vi "Auto-Fill.vi"() -> ()   [LabVIEW 2011]
uses:
  SubVI/Auto-Fill Cases.ctl
  SubVI/Valve_Pump.ctl
  SubVI/Pumps_Valves_Dependencies_Global.vi
panel:
  in  "Emergency Stop":bool
  out "Litres":dbl(slide) scale=0.0..14400.0
  out "Tank C":dbl(slide) scale=0.0..100.0
  out "Tank B":dbl(slide) scale=0.0..100.0
  out "Tank D":dbl(slide) scale=0.0..100.0
  out "Tank A":dbl(slide) scale=0.0..100.0
  in  "Density (kg/m3)":dbl[](array[numeric])=[0.0, 0.0, 0.0, 0.0, 0.0, 0.0]
  in  "Height (cm)":dbl[](array[numeric])=[0.0, 0.0, 0.0, 0.0, 0.0, 0.0]
  in  "Auto-Fill":T1
  in  "Start Process":bool
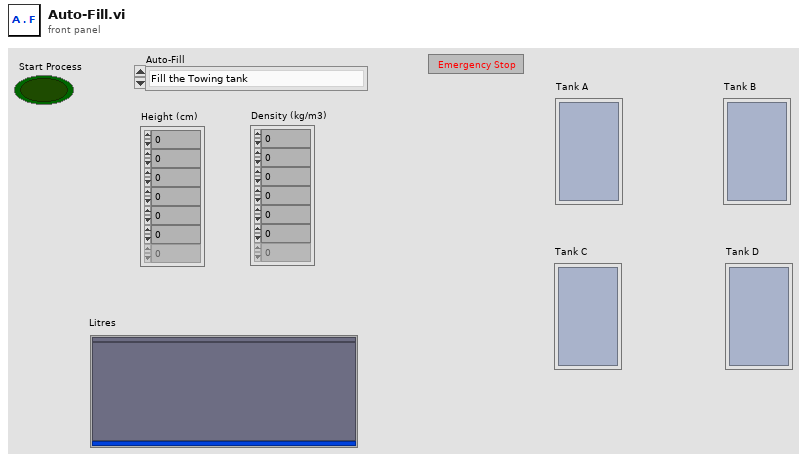
[diagram p1: front panel]
types:
  T1 = typedef "Auto-Fill Cases.ctl" = enum16{"Fill the Towing tank", "Fill Tank A from the Salt saturator tank", "Fill Tank B from the Salt Saturator tank", "Fill Tank C from the water mains", "Fill Tank D from the water mains", "Fill tank B from tank A", "Fill tank C from tank D"}
  T2 = typedef "Valve_Pump.ctl" = enum16{"Main Rack Power", "Pump Power", "Valve Power", "V4", "V5", "V6", "V7", "V8", "V9", "V10", "V11", "V12", "V13", "V14", "V15", "V18", "V19", "V20", "V21", "V22", "V23", "V24", "V25", "V26", "V27", "V28", "V29", "V30", "V31", "V32", "V33", "V34", "Pump A", "Pump B", "Pump C", "Pump D"}
  T3 = cluster{"Tanks[0]":dbl, "Tanks[1]":dbl, "Tanks[2]":dbl, "Tanks[3]":dbl, "Tanks[4]":dbl}
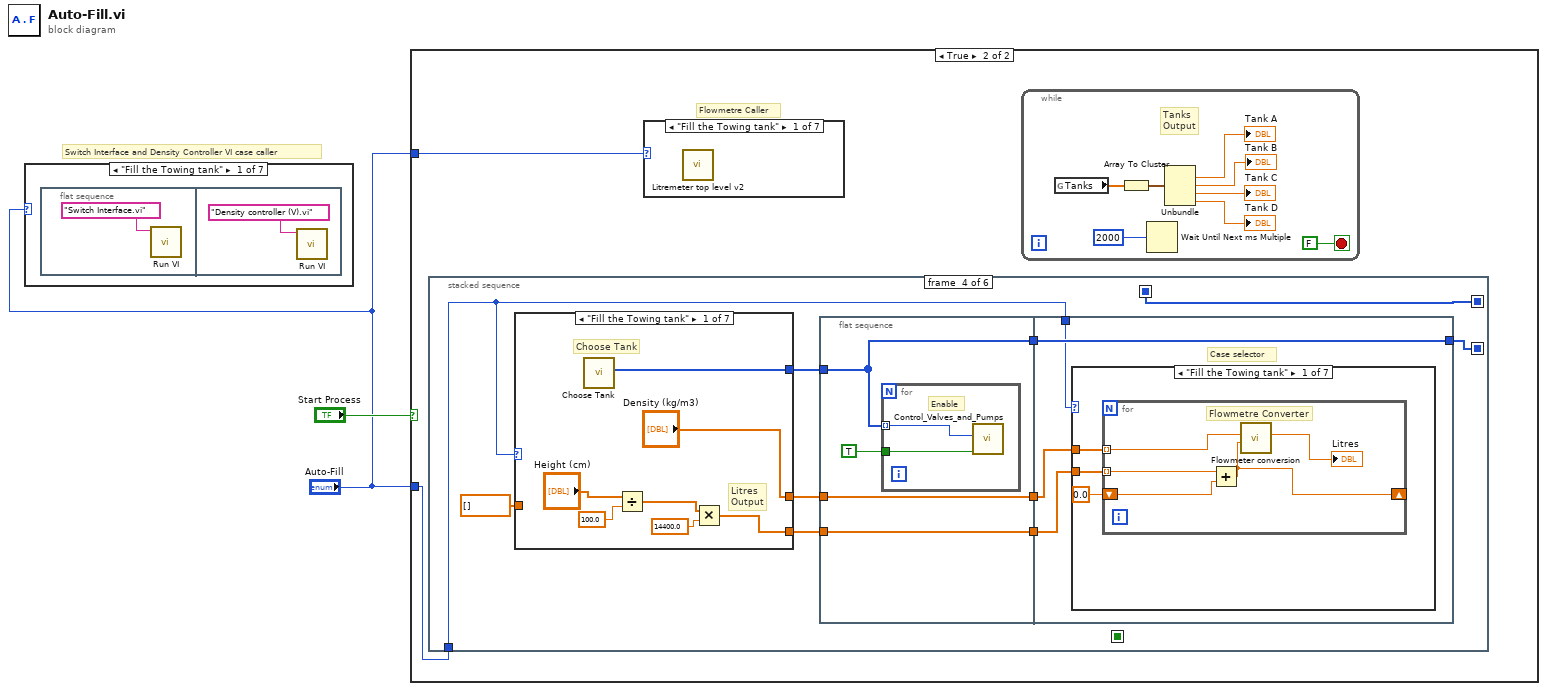
[diagram p0: block diagram]
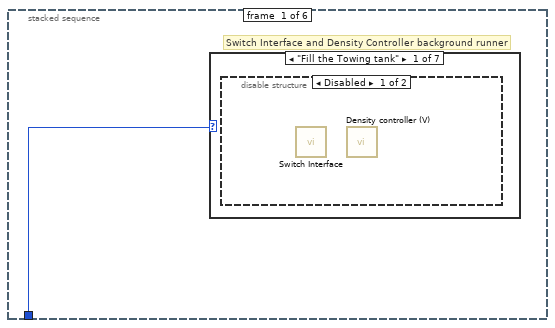
[diagram p15: hidden frame]
diagram:
  # "Switch Interface and Density Controller VI case caller"
  n1 = case shown="\"Fill the Towing tank\"" "Auto-Fill" {
    frame "Fill the Towing tank" {
      n2 = flat-sequence {
        frame #0 {
          n3 = call "Run VI.vi"("VI name"="Switch Interface.vi") -> ()  [unwired: 11 in]
        }
        frame #1 {
          n4 = call "Run VI.vi"("VI name"="Density controller (V).vi") -> ()  [unwired: 11 in]
        }
      }
    }
    frame "Fill Tank A from the Salt saturator tank" {
    }
    frame "Fill Tank B from the Salt Saturator tank" {
    }
    frame "Fill Tank C from the water mains" {
    }
    frame "Fill Tank D from the water mains" {
    }
    frame "Fill tank B from tank A" {
    }
    frame "Fill tank C from tank D" {
    }
  }
  n5 = case shown="True" "Start Process" {
    tunnel: "Auto-Fill" -> [_ w6]
    tunnel: "Auto-Fill" -> [_ w5]
    frame False {
    }
    frame True {
      # "Flowmetre Caller"
      n6 = stacked-sequence {
        seq-local: [_ _ w21 _ _ _] -> [_ _ _ w34 _ _]
        seq-local: [_ _ _ w31 _ _] -> [_ _ _ _ w141 _]
        seq-local: [_ _ _ w34 _ _] -> [_ _ _ _ w140 _]
        seq-local: [_ _ _ _ w137 _] -> [_ _ _ _ _ w145]
        tunnel: w6 -> [w15 _ _ w25 _ _]
        frame #0 {
          # "Switch Interface and Density Controller background runner"
          n7 = case shown="\"Fill the Towing tank\"" w15 {
            frame "Fill the Towing tank" {
              n8 = disable-structure shown="Disabled" {
                frame Disabled {
                  n9 = call "Switch Interface.vi"() -> ()  [unwired: 12 in]
                  n10 = call "Density controller (V).vi"() -> ()  [unwired: 12 in]
                }
                frame Enabled {
                }
              }
            }
            frame "Fill Tank A from the Salt saturator tank" {
            }
            frame "Fill Tank B from the Salt Saturator tank" {
            }
            frame "Fill Tank C from the water mains" {
            }
            frame "Fill Tank D from the water mains" {
            }
            frame "Fill tank B from tank A" {
            }
            frame "Fill tank C from tank D" {
            }
          }
        }
        frame #1 {
          # "Sequence delay time to allow Switch Interface VI to initialize"
          n11 = Wait (ms)(milliseconds to wait=u32 50000 ("millisecond multiple")) -> ()  [unwired: 1 out]
        }
        frame #2 {
          # "Identifier array\nbuild-up"
          n12 = Build Array(Valve_Pump."Main Rack Power" ("Device"), Valve_Pump."Pump Power" ("Device"), Valve_Pump."Valve Power" ("Device")) -> (w21:T2[])
          n13 = for {
            tunnel: TRUE -> [w23]
            tunnel: w21 -> [w24] mode=indexing
            # "Time delay"
            n14 = call "Control_Valves_and_Pumps.vi"("Set state:"=w23, "Device"=w24) -> ()  [unwired: 10 in]
            n15 = Wait Until Next ms Multiple(millisecond multiple=3000) -> ()  [unwired: 1 out]
          }
        }
        frame #3 {
          n16 = case shown="\"Fill the Towing tank\"" w25 {
            tunnel: [w107 w109 w114 w119 w122 w126 w132] -> w32
            tunnel: [w101 w108 w113 w118 w121 w124 w130] -> w26
            tunnel: ["Density (kg/m3)" w108 w113 w118 w121 w124 w130] -> w29
            tunnel: dbl[] [] ("Density (kg/m3)") -> [_ w108 w113 w118 w121 w124 w130]
            frame "Fill the Towing tank" {
              # "Choose Tank"
              # "Litres\nOutput"
              n17 = call "Choose Tank.vi"() -> ("Device"=w107:T2[])  [unwired: 9 in]
              n18 = Divide(x="Height (cm)", y=100.0) -> (x/y=w103:dbl[])
              n19 = Multiply(x=w103, y=14400.0) -> (x*y=w101:dbl[])
            }
            frame "Fill Tank A from the Salt saturator tank" {
              n20 = Build Array(Valve_Pump."V29" ("Device"), Valve_Pump."V27" ("Device"), Valve_Pump."Pump A" ("Device")) -> (w109:T2[])
            }
            frame "Fill Tank B from the Salt Saturator tank" {
              n21 = Build Array(Valve_Pump."V29" ("Device"), Valve_Pump."V23" ("Device"), Valve_Pump."Pump A" ("Device")) -> (w114:T2[])
            }
            frame "Fill Tank C from the water mains" {
              # "Identifier array\nbuild-up"
              n22 = Build Array(Valve_Pump."V8" ("Device")) -> (w119:T2[])
            }
            frame "Fill Tank D from the water mains" {
              # "Identifier array\nbuild-up"
              n23 = Build Array(Valve_Pump."V10" ("Device")) -> (w122:T2[])
            }
            frame "Fill tank B from tank A" {
              # "Identifier array\nbuild-up"
              n24 = Build Array(Valve_Pump."V4" ("Device"), Valve_Pump."V20" ("Device"), Valve_Pump."V22" ("Device"), Valve_Pump."Pump B" ("Device")) -> (w126:T2[])
            }
            frame "Fill tank C from tank D" {
              # "Identifier array\nbuild-up"
              n25 = Build Array(Valve_Pump."V9" ("Device"), Valve_Pump."V15" ("Device"), Valve_Pump."V20" ("Device"), Valve_Pump."V24" ("Device"), Valve_Pump."Pump B" ("Device")) -> (w132:T2[])
            }
          }
          n26 = flat-sequence {
            tunnel: [w37] -> w33
            tunnel: w32 -> [w37]
            tunnel: [w36] -> w30
            tunnel: w29 -> [w36]
            tunnel: [w35] -> w28
            tunnel: w26 -> [w35]
            tunnel: w33 -> [w44]
            tunnel: [w44] -> w31
            tunnel: w30 -> [w43]
            tunnel: w28 -> [w42]
            tunnel: w25 -> [w41]
            frame #0 {
              n27 = for {
                tunnel: w37 -> [w40] mode=indexing
                tunnel: TRUE -> [w39]
                # "Enable"
                n28 = call "Control_Valves_and_Pumps.vi"("Set state:"=w39, "Device"=w40) -> ()  [unwired: 10 in]
              }
            }
            frame #1 {
              # "Case selector"
              n29 = case shown="\"Fill the Towing tank\"" w41 {
                tunnel: w43 -> [w47 _ _ _ _ _ _]
                tunnel: w42 -> [w46 _ _ _ _ _ _]
                frame "Fill the Towing tank" {
                  n30 = for {
                    tunnel: w46 -> [w51] mode=indexing
                    tunnel: w47 -> [w52] mode=indexing
                    shift-right: [w50] -> _
                    shift-left: 0.0 -> [w49]
                    # "Flowmetre Converter"
                    n31 = Add(x=w51, y=w49) -> (x+y=w50:dbl)
                    n32 = call "Flowmeter conversion.vi"("Required Litres"=w50, "Density Required"=w52) -> ("Total Litres (calc)"=→"Litres":dbl)  [unwired: 9 in]
                  }
                }
                frame "Fill Tank A from the Salt saturator tank" {
                  n33 = while {
                    stop <- w55 continue-if-true
                    n34 = flat-sequence {
                      tunnel: [w58] -> w56
                      frame #0 {
                        n35 = call "Tank height conversion.vi"() -> ()  [unwired: 11 in, 1 out]
                      }
                      frame #1 {
                        # "Full case checker"
                        n36 = global read "Pumps_Valves_Dependencies_Global.vi" "Tank A"() -> (w60:dbl)
                        n37 = Less?(x=w60, y=90.0) -> (x < y?=w58:bool)
                      }
                    }
                    n38 = Wait Until Next ms Multiple(millisecond multiple=2000) -> ()  [unwired: 1 out]
                    n39 = local read "Emergency Stop"() -> (w53:bool)
                    n40 = Not(x=w53) -> (.not. x?=w54:bool)
                    n41 = And(x=w56, y=w54) -> (x .and. y?=w55:bool)
                  }
                }
                frame "Fill Tank B from the Salt Saturator tank" {
                  n42 = while {
                    stop <- w63 continue-if-true
                    n43 = flat-sequence {
                      tunnel: [w67] -> w64
                      frame #0 {
                        n44 = call "Tank height conversion.vi"() -> ()  [unwired: 11 in, 1 out]
                      }
                      frame #1 {
                        # "Full case checker"
                        n45 = global read "Pumps_Valves_Dependencies_Global.vi" "Tank B"() -> (w66:dbl)
                        n46 = Less?(x=w66, y=80.0) -> (x < y?=w67:bool)
                      }
                    }
                    n47 = Wait Until Next ms Multiple(millisecond multiple=2000) -> ()  [unwired: 1 out]
                    n48 = local read "Emergency Stop"() -> (w61:bool)
                    n49 = Not(x=w61) -> (.not. x?=w62:bool)
                    n50 = And(x=w64, y=w62) -> (x .and. y?=w63:bool)
                  }
                }
                frame "Fill Tank C from the water mains" {
                  n51 = while {
                    stop <- w71 continue-if-true
                    n52 = flat-sequence {
                      tunnel: [w74] -> w72
                      frame #0 {
                        n53 = call "Tank height conversion.vi"() -> ()  [unwired: 11 in, 1 out]
                      }
                      frame #1 {
                        # "Full case checker"
                        n54 = global read "Pumps_Valves_Dependencies_Global.vi" "Tank C"() -> (w76:dbl)
                        n55 = Less?(x=w76, y=90.0) -> (x < y?=w74:bool)
                      }
                    }
                    n56 = Wait Until Next ms Multiple(millisecond multiple=2000) -> ()  [unwired: 1 out]
                    n57 = Not(x="Emergency Stop") -> (.not. x?=w70:bool)
                    n58 = And(x=w72, y=w70) -> (x .and. y?=w71:bool)
                  }
                }
                frame "Fill Tank D from the water mains" {
                  n59 = while {
                    stop <- w79 continue-if-true
                    n60 = flat-sequence {
                      tunnel: [w82] -> w80
                      frame #0 {
                        n61 = call "Tank height conversion.vi"() -> ()  [unwired: 11 in, 1 out]
                      }
                      frame #1 {
                        # "Full case checker"
                        n62 = global read "Pumps_Valves_Dependencies_Global.vi" "Tank D"() -> (w84:dbl)
                        n63 = Less?(x=w84, y=90.0) -> (x < y?=w82:bool)
                      }
                    }
                    n64 = Wait Until Next ms Multiple(millisecond multiple=2000) -> ()  [unwired: 1 out]
                    n65 = local read "Emergency Stop"() -> (w77:bool)
                    n66 = Not(x=w77) -> (.not. x?=w78:bool)
                    n67 = And(x=w80, y=w78) -> (x .and. y?=w79:bool)
                  }
                }
                frame "Fill tank B from tank A" {
                  n68 = while {
                    stop <- w87 continue-if-true
                    n69 = flat-sequence {
                      tunnel: [w90] -> w88
                      frame #0 {
                        n70 = call "Tank height conversion.vi"() -> ()  [unwired: 11 in, 1 out]
                      }
                      frame #1 {
                        # "Full case checker"
                        n71 = global read "Pumps_Valves_Dependencies_Global.vi" "Tank B"() -> (w92:dbl)
                        n72 = Less?(x=w92, y=90.0) -> (x < y?=w90:bool)
                      }
                    }
                    n73 = Wait Until Next ms Multiple(millisecond multiple=2000) -> ()  [unwired: 1 out]
                    n74 = local read "Emergency Stop"() -> (w85:bool)
                    n75 = Not(x=w85) -> (.not. x?=w86:bool)
                    n76 = And(x=w88, y=w86) -> (x .and. y?=w87:bool)
                  }
                }
                frame "Fill tank C from tank D" {
                  n77 = while {
                    stop <- w95 continue-if-true
                    n78 = flat-sequence {
                      tunnel: [w98] -> w96
                      frame #0 {
                        n79 = call "Tank height conversion.vi"() -> ()  [unwired: 11 in, 1 out]
                      }
                      frame #1 {
                        # "Full case checker"
                        n80 = global read "Pumps_Valves_Dependencies_Global.vi" "Tank C"() -> (w100:dbl)
                        n81 = Less?(x=w100, y=90.0) -> (x < y?=w98:bool)
                      }
                    }
                    n82 = Wait Until Next ms Multiple(millisecond multiple=2000) -> ()  [unwired: 1 out]
                    n83 = local read "Emergency Stop"() -> (w94:bool)
                    n84 = Not(x=w94) -> (.not. x?=w93:bool)
                    n85 = And(x=w96, y=w93) -> (x .and. y?=w95:bool)
                  }
                }
              }
            }
          }
        }
        frame #4 {
          w137 = FALSE ("Set state:")
          # "Identifier array inverse\nbuild-up"
          n86 = Build Array (concatenate)(w140, w141) -> (w139:T2[])
          n87 = Reverse 1D Array(array=w139) -> (reversed array=w138:T2[])
          n88 = for {
            tunnel: w137 -> [w144]
            tunnel: w138 -> [w143] mode=indexing
            # "Time delay"
            n89 = call "Control_Valves_and_Pumps.vi"("Set state:"=w144, "Device"=w143) -> ()  [unwired: 10 in]
            n90 = Wait Until Next ms Multiple(millisecond multiple=5000) -> ()  [unwired: 1 out]
          }
        }
        frame #5 {
          n91 = local write "Start Process"(w145) -> ()
        }
      }
      n92 = case shown="\"Fill the Towing tank\"" w5 {
        frame "Fill the Towing tank" {
          n93 = call "Litremeter top level v2.vi"() -> ()  [unwired: 1 in]
        }
        frame "Fill Tank A from the Salt saturator tank" {
        }
        frame "Fill Tank B from the Salt Saturator tank" {
        }
        frame "Fill Tank C from the water mains" {
        }
        frame "Fill Tank D from the water mains" {
        }
        frame "Fill tank B from tank A" {
        }
        frame "Fill tank C from tank D" {
        }
      }
      n94 = while {
        stop <- FALSE stop-if-true
        # "Tanks \nOutput"
        n95 = global read "Pumps_Valves_Dependencies_Global.vi" "Tanks"() -> (w13:dbl[])
        n96 = Array To Cluster(array=w13) -> (cluster=w14:T3)
        n97 = Wait Until Next ms Multiple(millisecond multiple=2000) -> ()  [unwired: 1 out]
        n98 = Unbundle(w14) -> ("Tanks[1]"=→"Tank A":dbl, "Tanks[2]"=→"Tank B":dbl, "Tanks[3]"=→"Tank C":dbl, "Tanks[4]"=→"Tank D":dbl)  [unwired: 1 out]
      }
    }
  }
